vi "main.vi"   [LabVIEW 2021]
uses:
  Control Property Tree/Control Property Tree.lvlib
  Libraries/Property Panel Launcher/Property Panel Launcher.lvlib
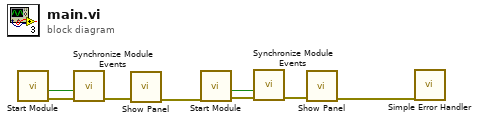
[diagram p0: block diagram]
diagram:
  n1 = call "Start Module.vi"() -> ("error out"=w7:errorcluster, "Wait for Event Sync?"=w8:bool)  [unwired: 8 in, 2 out]
  n2 = call "Synchronize Module Events.vi"("error in (no error)"=w7, "Wait for Event Sync?"=w8) -> ("error out"=w4:errorcluster)  [unwired: 9 in]
  n3 = call "Show Panel.vi"("error in (no error)"=w4) -> ("error out"=w1:errorcluster)  [unwired: 10 in]
  n4 = call "Start Module.vi"("error in (no error)"=w1) -> ("error out"=w5:errorcluster, "Wait for Event Sync?"=w6:bool)  [unwired: 7 in, 2 out]
  n5 = call "Synchronize Module Events.vi"("error in (no error)"=w5, "Wait for Event Sync?"=w6) -> ("error out"=w3:errorcluster)  [unwired: 9 in]
  n6 = call "Show Panel.vi"("error in (no error)"=w3) -> ("error out"=w2:errorcluster)  [unwired: 10 in]
  n7 = call <vilib>:"Simple Error Handler.vi"("error in (no error)"=w2) -> ()  [unwired: 4 in, 5 out]
